vi "Get RTD Props.vi"(8 "error in (no error)":errorcluster, 11 "Item Ref in":T2 format="%.0x") -> (0 "error out":errorcluster, 2 "temp param":T1={"A"=0.00139999995008111, "B"=0.00023700000019744039, "C"=9.899999753315569e-08, "R0"=1000.0}, 3 "Item Ref out":T2 format="%.0x")   [LabVIEW 2011, in "NI 272x Resistive Simulation Custom Device Configuration.lvlib"]
uses:
  NI 272x Resistive Simulation Custom Device Configuration.lvlib
  <vilib>/NI Veristand/Custom Device API/Custom Device Item Ref.ctl
  <instrlib>/ni272xReferenceVIs/ni272xReferenceVIs.llb/ni272x Callendar-Van Dusen RTD Parameters.ctl
  Globals/Names.vi
  <vilib>/NI Veristand/Custom Device API/Get Item Property (Double).vi
  NI 272x Resistive Simulation Custom Device Shared.lvlib
  <vilib>/NI Veristand/Custom Device API/Custom Device API.lvlib
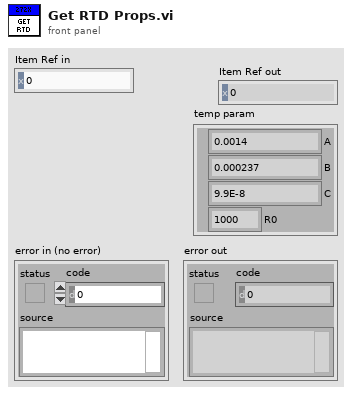
[diagram p1: front panel]
types:
  T1 = typedef "ni272x Callendar-Van Dusen RTD Parameters.ctl" = cluster{"A":dbl, "B":dbl, "C":dbl, "R0":dbl}
  T2 = typedef "Custom Device API.lvlib/Custom Device Item Ref.ctl" = u64
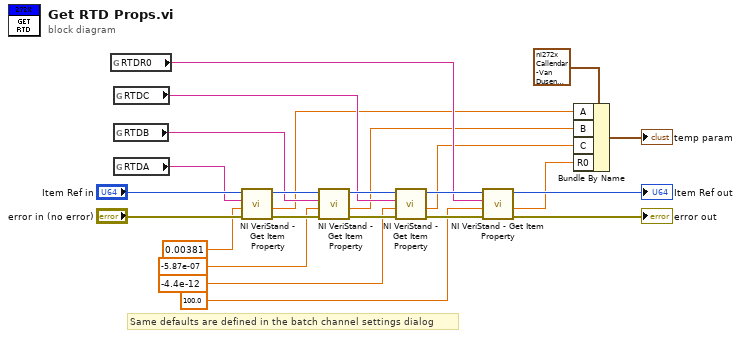
[diagram p0: block diagram]
diagram:
  # "Same defaults are defined in the batch channel settings dialog"
  n1 = global read "Names.vi" "RTDR0"() -> (w14:string)
  n2 = global read "Names.vi" "RTDC"() -> (w15:string)
  n3 = global read "Names.vi" "RTDB"() -> (w16:string)
  n4 = global read "Names.vi" "RTDA"() -> (w22:string)
  n5 = call-poly <vilib>:"NI VeriStand - Get Item Property.vi"("error in (no error)"="error in (no error)", "Default Value"=0.00381 ("A"), "Property Name"=w22, "Item Ref in"="Item Ref in") -> ("error out"=w13:errorcluster, "Value"=w5:dbl, "Item Ref out"=w21:T2)  [unwired: 4 in, 1 out]
  n6 = call-poly <vilib>:"NI VeriStand - Get Item Property.vi"("error in (no error)"=w13, "Default Value"=-5.87e-07 ("B"), "Property Name"=w16, "Item Ref in"=w21) -> ("error out"=w12:errorcluster, "Value"=w4:dbl, "Item Ref out"=w20:T2)  [unwired: 4 in, 1 out]
  n7 = call-poly <vilib>:"NI VeriStand - Get Item Property.vi"("error in (no error)"=w12, "Default Value"=-4.4e-12 ("C"), "Property Name"=w15, "Item Ref in"=w20) -> ("error out"=w11:errorcluster, "Value"=w3:dbl, "Item Ref out"=w19:T2)  [unwired: 4 in, 1 out]
  n8 = call-poly <vilib>:"NI VeriStand - Get Item Property.vi"("error in (no error)"=w11, "Default Value"=100.0 ("R0"), "Property Name"=w14, "Item Ref in"=w19) -> ("error out"=→"error out":errorcluster, "Value"=w2:dbl, "Item Ref out"=→"Item Ref out":T2)  [unwired: 4 in, 1 out]
  n9 = Bundle By Name(cluster=T1 {"A"=0.00139999995008111, "B"=0.00023700000019744039, "C"=9.899999753315569e-08, "R0"=1000.0} ("temp param"), "A"=w5, "B"=w4, "C"=w3, "R0"=w2) -> (→"temp param":T1)
